vi "Generate Report from Templete(Word).vi"(9 "Graph":dbl[][](array[numeric])=[[1.0, 3.0], [2.0, 8.0], [3.0, 5.0]] format="%.2f", 11 "error in (no error)":errorcluster) -> (15 "error out":errorcluster)   [LabVIEW 2020]
uses:
  <vilib>/Utility/NIReport.llb/Append Report Text (str wrap).vi
  <vilib>/Utility/NIReport.llb/NI_report.lvclass
  <vilib>/Utility/NIReport.llb/Word/NI_Word.lvclass
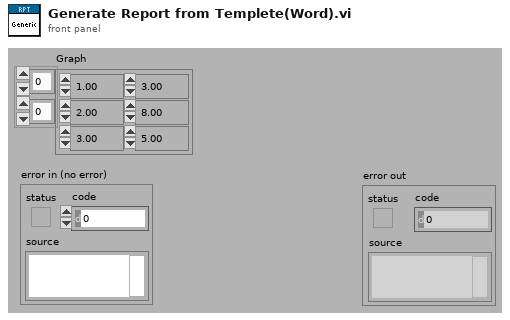
[diagram p1: front panel]
types:
  T1 = cluster{"position (Excel)":cluster{"row":i32, "column":i32}, "name (Excel)":string, "bookmark (Word)":string}
  T2 = enum16{"Standard Report", "HTML", "Word", "Excel"}
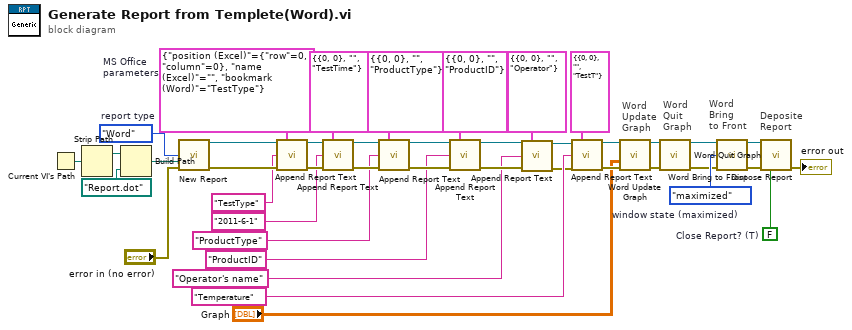
[diagram p0: block diagram]
diagram:
  w32 = FALSE  # Close Report? (T)
  w37 = enum16{"maximized", "minimized", "normal"}."maximized"  # window state (maximized)
  w41 = T1 {"position (Excel)"={"row"=0, "column"=0}, "name (Excel)"="", "bookmark (Word)"="TestType"}  # MS Office parameters
  w42 = T2."Word"  # report type
  # "Deposite\nReport"
  # "Word\nBring\nto Front"
  # "Word\nQuit\nGraph"
  # "Word\nUpdate\nGraph"
  n1 = Current VI's Path() -> (path=w5:path)
  n2 = Strip Path(path=w5) -> (stripped path=w4:path)  [unwired: 1 out]
  n3 = Build Path(base path=w4, name or relative path=path "Report.dot" ("template")) -> (appended path=w3:path)
  n4 = call <vilib>:"New Report.vi"("report type"=w42, "template (empty)"=w3, "error in (no error)"="error in (no error)") -> ("report out"=w29:refnum<class "NI_report.lvclass">, "error out"=w28:errorcluster)  [unwired: 11 in]
  n5 = call-poly <vilib>:"Append Report Text.vi"("report in"=w29, "MS Office parameters"=w41, "text"="TestType" ("TestType"), "error in (no error)"=w28) -> ("report out"=w31:refnum<class "NI_report.lvclass">, "error out"=w30:errorcluster)  [unwired: 8 in, 2 out]
  n6 = call-poly <vilib>:"Append Report Text.vi"("report in"=w31, "MS Office parameters"=T1 {"position (Excel)"={"row"=0, "column"=0}, "name (Excel)"="", "bookmark (Word)"="TestTime"}, "text"="2011-6-1" ("TestTime"), "error in (no error)"=w30) -> ("report out"=w25:refnum<class "NI_report.lvclass">, "error out"=w24:errorcluster)  [unwired: 8 in, 2 out]
  n7 = call-poly <vilib>:"Append Report Text.vi"("report in"=w25, "MS Office parameters"=T1 {"position (Excel)"={"row"=0, "column"=0}, "name (Excel)"="", "bookmark (Word)"="ProductType"}, "text"="ProductType" ("ProductType"), "error in (no error)"=w24) -> ("report out"=w26:refnum<class "NI_report.lvclass">, "error out"=w27:errorcluster)  [unwired: 8 in, 2 out]
  n8 = call-poly <vilib>:"Append Report Text.vi"("report in"=w26, "MS Office parameters"=T1 {"position (Excel)"={"row"=0, "column"=0}, "name (Excel)"="", "bookmark (Word)"="ProductID"}, "text"="ProductID" ("ProductID"), "error in (no error)"=w27) -> ("report out"=w21:refnum<class "NI_report.lvclass">, "error out"=w22:errorcluster)  [unwired: 8 in, 2 out]
  n9 = call-poly <vilib>:"Append Report Text.vi"("report in"=w21, "MS Office parameters"=T1 {"position (Excel)"={"row"=0, "column"=0}, "name (Excel)"="", "bookmark (Word)"="Operator"}, "text"="Operator's name" ("Operator"), "error in (no error)"=w22) -> ("report out"=w1:refnum<class "NI_report.lvclass">, "error out"=w2:errorcluster)  [unwired: 8 in, 2 out]
  n10 = call-poly <vilib>:"Append Report Text.vi"("report in"=w1, "MS Office parameters"=T1 {"position (Excel)"={"row"=0, "column"=0}, "name (Excel)"="", "bookmark (Word)"="TestT"}, "text"="Temperature" ("TestT"), "error in (no error)"=w2) -> ("report out"=w9:refnum<class "NI_report.lvclass">, "error out"=w10:errorcluster)  [unwired: 8 in, 2 out]
  n11 = call <vilib>:"Word Update Graph.vi"("report in"=w9, "graph data"="Graph", "error in (no error)"=w10) -> ("report out"=w39:refnum<class "NI_report.lvclass">, "error out"=w38:errorcluster)  [unwired: 11 in]
  n12 = call <vilib>:"Word Quit Graph.vi"("report in"=w39, "error in (no error)"=w38) -> ("report out"=w35:refnum<class "NI_report.lvclass">, "error out"=w36:errorcluster)  [unwired: 12 in]
  n13 = call <vilib>:"Word Bring to Front.vi"("report in"=w35, "window state (maximized)"=w37, "error in (no error)"=w36) -> ("report out"=w33:refnum<class "NI_report.lvclass">, "error out"=w34:errorcluster)  [unwired: 11 in]
  n14 = call-dynamic "Dispose Report.vi"("report in"=w33, "error in (no error)"=w34, "close report? (T)"=w32) -> ("error out"=→"error out":errorcluster)  [unwired: 12 in]
